vi "解析参数.vi"(0 "输入字符串":string="+RECW0Ú\u00046½Ö\u000f000\u000b\u0015†x6u_\u000b\u0013€\b\u0012P\u000f013<\u0000<\u0000<\u00000\rwww.baidu.comÿÿÿÿÿÿÿÿÿÿÿÿÿÿÿÿÿÿ\u0005CMNETÿÿÿÿÿÿÿÿÿÿÿÿÿÿÿÿÿÿÿÿÿÿÿÿÿÿ1\u000b\u0015†x5”O\u0000ÿÿÿÿÿÿ\u0000ÿÿÿÿÿÿÿÿÿÿÿÿÿÿÿD…") -> (1 "GPRS参数（TXJT）":T1={"IP地址"="192.168.1.1", "工作模式"=48, "连接协议"=48, "本机号码"="13806871122", "短信监控中心号码1"="13800577500", "监听时间"=0, "心跳间隔"=0, "重启时间(分)"=0, "C/S关系"=48, "DNS域名"="", "APN接入点"="", "报头使能"=48, "波特率"=45060, "短信目标号码1 "="", "短信目标号码2"="", "短信监控中心号码2"="", "信号检测使能"=48, "控制方式"=48, "端口号"=5070, "连接方式"=48} {"连接方式" items=["固定IP"=48, "域名解析"=49]; "控制方式" items=["软件控制"=48, "EN控制"=49]; "信号检测使能" items=["不检测"=48, "检测"=49]; "波特率" items=["1200"=51, "2400"=52, "4800"=48, "9600"=49, "19200"=50]; "报头使能" items=["上传"=48, "不上传"=49]; "C/S关系" items=["客服端"=48, "服务端"=49]; "连接协议" items=["TCP协议"=48, "UDP协议"=49]; "工作模式" items=["GPRS模式"=48, "短信模式"=49]}, 2 "字符串":string, 3 "参数是否获取":bool=TRUE)   [LabVIEW 2015]
panel:
  out "波特率 4":u16
  in  "波特率 2":u16(ring)=45060 items=["1200"=81, "2400"=82, "4800"=72, "9600"=73, "19200"=80]
  out "长度":i32
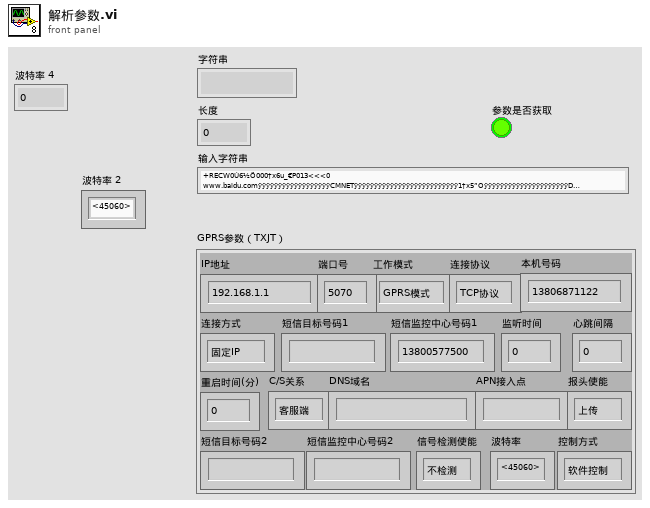
[diagram p1: front panel]
types:
  T1 = typedef "GPRS参数DW02.ctl" = cluster{"IP地址":string, "工作模式":u16, "连接协议":u16, "本机号码":string, "短信监控中心号码1":string, "监听时间":u16, "心跳间隔":u16, "重启时间(分)":u16, "C/S关系":u16, "DNS域名":string, "APN接入点":string, "报头使能":u16, "波特率":u16, "短信目标号码1 ":string, "短信目标号码2":string, "短信监控中心号码2":string, "信号检测使能":u16, "控制方式":u16, "端口号":u16, "连接方式":u16}
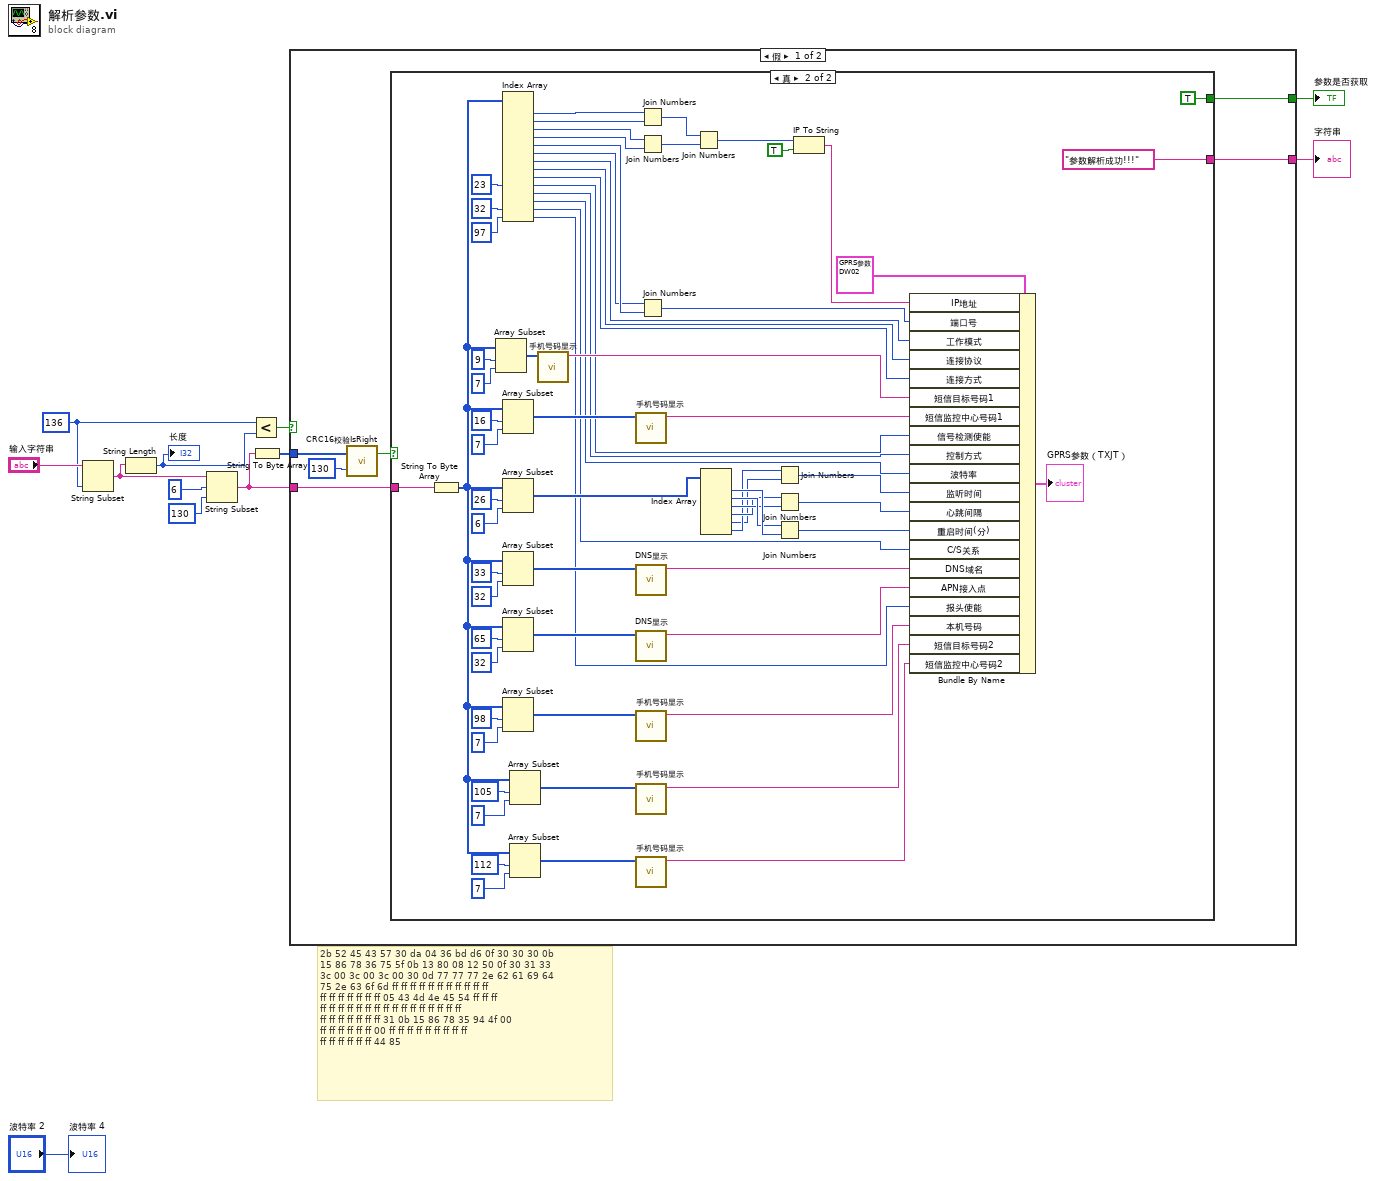
[diagram p0: block diagram]
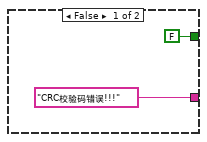
[diagram p2: hidden frame]
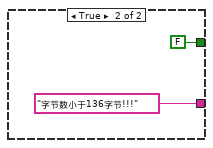
[diagram p3: hidden frame]
diagram:
  w2 = 136 ("x")
  # "2b 52 45 43 57 30 da 04 36 bd d6 0f 30 30 30 0b \n15 86 78 36 75 5f 0b 13 80 08 12 50 0f 30 31 33 \n3c 00 3c 00 3c 00 30 0d 77 77 77 2e 62 61 69 64 \n75 2e 63 6f 6d ff ff ff ff ff ff ff ff ff ff ff \nff ff ff ff ff ff ff 05 43 4d 4e 45 54 ff ff ff \nff ff ff ff ff ff ff ff ff ff ff ff ff ff ff ff \nff ff ff ff ff ff ff 31 0b 15 86 78 35 94 4f 00 \nff ff ff ff ff ff 00 ff ff ff ff ff ff ff ff ff \nff ff ff ff ff ff 44 85"
  n1 = String Subset(string="输入字符串", length (rest)=w2) -> (substring=w3:string)  [unwired: 1 in]
  n2 = String Length(string=w3) -> (length=w12:i32)
  "长度" <- w12
  n3 = String Subset(string=w3, offset (0)=6 ("偏移量(0)"), length (rest)=130 ("长度（剩余）")) -> (substring=w7:string)
  n4 = Less?(x=w2, y=w12) -> (x < y?=w11:bool)
  n5 = String To Byte Array(string=w7) -> (unsigned byte array=w10:u8[])
  n6 = case shown="假" w11 {
    tunnel: w10 -> [w18 _]
    tunnel: w7 -> [w15 _]
    tunnel: [w14 "字节数小于136字节!!!" ("输入字符串 2")] -> w6
    tunnel: [w13 FALSE ("参数是否获取 2")] -> w5
    frame False {
      n7 = call "CRC16校验IsRight.vi"("含检验码数据长度"=u16 130, "输入数据"=w18) -> ("布尔"=w16:bool)  [unwired: 1 out]
      n8 = case shown="真" w16 {
        tunnel: w15 -> [_ w87]
        tunnel: [FALSE ("参数是否获取 2") TRUE ("参数是否获取 2")] -> w13
        tunnel: ["CRC校验码错误!!!" ("输入字符串 2") "参数解析成功!!!" ("字符串 2")] -> w14
        frame False {
        }
        frame True {
          n9 = String To Byte Array(string=w87) -> (unsigned byte array=w89:u8[])
          n10 = Array Subset(array=w89, index=9 ("索引"), length=7 ("长度")) -> (w67:u8[])
          n11 = Index Array(array=w89, index #10=23 ("索引"), index #13=32 ("索引"), index #14=97 ("索引")) -> (element #1=w85:u8, element #2=w84:u8, element #3=w83:u8, element #4=w82:u8, element #5=w76:u8, element #6=w75:u8, element #7=w73:u8, element #8=w72:u8, element #9=w71:u8, element #10=w32:u8, element #11=w31:u8, element #12=w21:u8, element #13=w30:u8, element #14=w28:u8)  [unwired: 11 in]
          n12 = Array Subset(array=w89, index=16 ("索引"), length=7 ("长度")) -> (w64:u8[])
          n13 = Array Subset(array=w89, index=26 ("索引"), length=6 ("长度")) -> (w60:u8[])
          n14 = Array Subset(array=w89, index=33 ("索引"), length=32 ("长度")) -> (w50:u8[])
          n15 = Array Subset(array=w89, index=65 ("索引"), length=32 ("长度")) -> (w47:u8[])
          n16 = Array Subset(array=w89, index=98 ("索引"), length=7 ("长度")) -> (w43:u8[])
          n17 = Array Subset(array=w89, index=105 ("索引"), length=7 ("长度")) -> (w40:u8[])
          n18 = Array Subset(array=w89, index=112 ("索引"), length=7 ("长度")) -> (w38:u8[])
          n19 = call "手机号码显示.vi"("手机号码内容"=w67) -> ("字符串"=w68:string)  [unwired: 10 in]
          n20 = call "手机号码显示.vi"("手机号码内容"=w64) -> ("字符串"=w63:string)  [unwired: 10 in]
          n21 = call "DNS显示.vi"("DNS数组"=w50) -> ("输出显示"=w49:string)  [unwired: 10 in]
          n22 = call "DNS显示.vi"("DNS数组"=w47) -> ("输出显示"=w48:string)  [unwired: 10 in]
          n23 = call "手机号码显示.vi"("手机号码内容"=w43) -> ("字符串"=w42:string)  [unwired: 10 in]
          n24 = call "手机号码显示.vi"("手机号码内容"=w40) -> ("字符串"=w39:string)  [unwired: 10 in]
          n25 = call "手机号码显示.vi"("手机号码内容"=w38) -> ("字符串"=w37:string)  [unwired: 10 in]
          n26 = Join Numbers(hi=w85, lo=w84) -> ((hi.lo)=w81:u16)
          n27 = Join Numbers(hi=w83, lo=w82) -> ((hi.lo)=w80:u16)
          n28 = Join Numbers(hi=w75, lo=w76) -> ((hi.lo)=w74:u16)
          n29 = Join Numbers(hi=w81, lo=w80) -> ((hi.lo)=w79:u32)
          n30 = Index Array(array=w60) -> (element #1=w59:u8, element #2=w58:u8, element #3=w57:u8, element #4=w56:u8, element #5=w54:u8, element #6=w55:u8)  [unwired: 6 in]
          n31 = Join Numbers(hi=w55, lo=w54) -> ((hi.lo)=w24:u16)
          n32 = Join Numbers(hi=w56, lo=w57) -> ((hi.lo)=w25:u16)
          n33 = Join Numbers(hi=w58, lo=w59) -> ((hi.lo)=w26:u16)
          n34 = IP To String(1:TRUE ("句点符号？(F)"), 2:w79) -> (0:w77:string)
          n35 = Bundle By Name(cluster=T1 {"IP地址"="000.000.000.000", "工作模式"=48, "连接协议"=48, "本机号码"="13806871122", "短信监控中心号码1"="13800577500", "监听时间"=10000, "心跳间隔"=0, "重启时间(分)"=0, "C/S关系"=49, "DNS域名"="", "APN接入点"="", "报头使能"=49, "波特率"=81, "短信目标号码1 "="", "短信目标号码2"="", "短信监控中心号码2"="", "信号检测使能"=48, "控制方式"=48, "端口号"=50700, "连接方式"=49} ("GPRS参数（TXJT） 2"), "IP地址"=w77, "端口号"=w74, "工作模式"=w73, "连接协议"=w72, "连接方式"=w71, "短信目标号码1"=w68, "短信监控中心号码1"=w63, "信号检测使能"=w32, "控制方式"=w31, "波特率"=w21, "监听时间"=w24, "心跳间隔"=w25, "重启时间(分)"=w26, "C/S关系"=w30, "DNS域名"=w49, "APN接入点"=w48, "报头使能"=w28, "本机号码"=w42, "短信目标号码2"=w39, "短信监控中心号码2"=w37) -> (→"GPRS参数（TXJT）":T1)
        }
      }
    }
    frame True {
    }
  }
  "字符串" <- w6
  "参数是否获取" <- w5
  "波特率 4" <- "波特率 2"
